vi "MT_write4.vi"(7 "duration":dbl, 8 "error in":errorcluster, 9 "sampling rate":dbl, 10 "samples per channel":i32=1000, 11 "data":dbl[][](array[numeric]) format="%0.2f") -> (0 "error out":errorcluster)   [LabVIEW 2019]
uses:
  <vilib>/DAQmx/write.llb/DAQmx Write (Analog 2D DBL NChan NSamp).vi
  <vilib>/DAQmx/create/channels.llb/DAQmx Create Channel (AO-Voltage-Basic).vi
  <vilib>/DAQmx/configure/timing.llb/DAQmx Timing (Sample Clock).vi
  <vilib>/DAQmx/miscellaneous.llb/DAQmx Fill In Error Info.vi
panel:
  in  "stop":bool
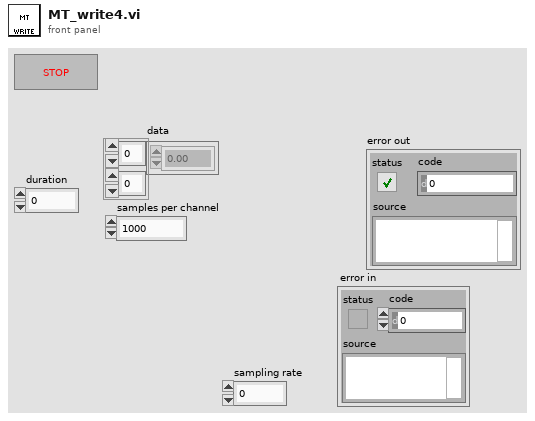
[diagram p1: front panel]
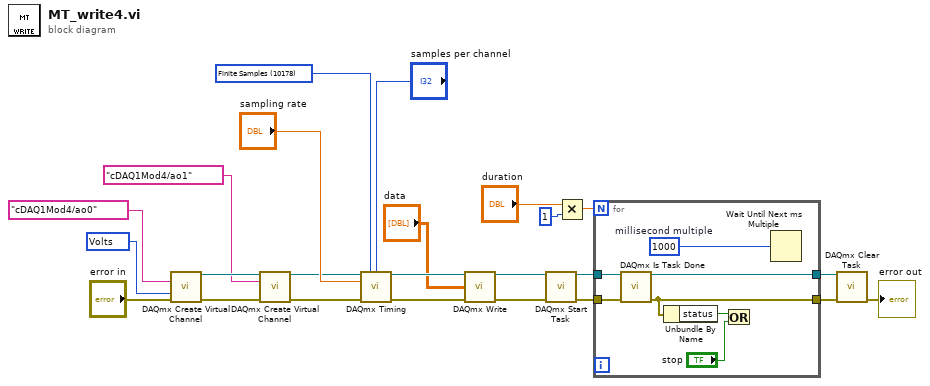
[diagram p0: block diagram]
diagram:
  w18 = 10348 items=["Volts"=10348, "From Custom Scale"=10065] ("units")
  w21 = 10178 items=["Finite Samples"=10178, "Continuous Samples"=10123] ("sample mode")
  n1 = call-poly <vilib>:"DAQmx Create Virtual Channel.vi"("physical channels"=tag "cDAQ1Mod4/ao0", "units"=w18, "error in"="error in") -> ("task out"=w16:refnum<k21>, "error out"=w15:errorcluster)  [unwired: 6 in, 5 out]
  n2 = call-poly <vilib>:"DAQmx Create Virtual Channel.vi"("task in"=w16, "physical channels"=tag "cDAQ1Mod4/ao1", "error in"=w15) -> ("task out"=w14:refnum<k21>, "error out"=w13:errorcluster)  [unwired: 11 in]
  n3 = call-poly <vilib>:"DAQmx Timing.vi"("task/channels in"=w14, "sample mode"=w21, "samples per channel"="samples per channel", "rate"="sampling rate", "error in"=w13) -> ("task out"=w22:refnum<k21>, "error out"=w23:errorcluster)  [unwired: 2 in, 7 out]
  n4 = call-poly <vilib>:"DAQmx Write.vi"("task/channels in"=w22, "data"="data", "error in"=w23) -> ("task out"=w4:refnum<k21>, "error out"=w5:errorcluster)  [unwired: 1 in, 10 out]
  n5 = call <vilib>:"DAQmx Start Task.vi"("task/channels in"=w4, "error in"=w5) -> ("task out"=w6:refnum<k21>, "error out"=w7:errorcluster)  [unwired: 12 out]
  n6 = Multiply(x="duration", y=1) -> (x*y=w9:dbl)
  n7 = for {
    N: w9 -> [_]
    tunnel: w6 -> [w31]
    tunnel: [w30] -> w3
    tunnel: w7 -> [w29]
    tunnel: [w27] -> w2
    w25 = u32 1000  # millisecond multiple
    n8 = call <vilib>:"DAQmx Is Task Done.vi"("task/channels in"=w31, "error in"=w29) -> ("task out"=w30:refnum<k21>, "error out"=w27:errorcluster)  [unwired: 1 in, 11 out]
    n9 = Unbundle By Name(w27) -> ("status"=w28:bool)
    n10 = Or(x=w28, y="stop") -> ()  [unwired: 1 out]
    n11 = Wait Until Next ms Multiple(millisecond multiple=w25) -> ()  [unwired: 1 out]
  }
  n12 = call <vilib>:"DAQmx Clear Task.vi"("task in"=w3, "error in"=w2) -> ("error out"=→"error out":errorcluster)  [unwired: 13 out]
